vi "UAPublishNode.vi"(8 "error in (no error)":errorcluster, 9 "parent opcua path":string, 10 "OPC UA server refnum in":refnum<k21>, 11 "content":string) -> (0 "error out":errorcluster, 2 "OPC UA server refnum out":refnum<k21>)   [LabVIEW 2014, in "OPCUA XML(dev).lvlib"]
uses:
  OPCUA XML(dev).lvlib
  <vilib>/regexp/Match Regular Expression.xnode
  <vilib>/OPCUA/NI OPC UA Server.lvlib
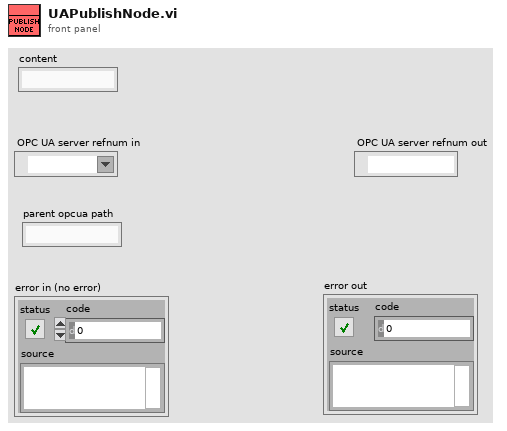
[diagram p1: front panel]
types:
  T1 = cluster{"name":string, "data type":u16, "access level":u16, "description":string}
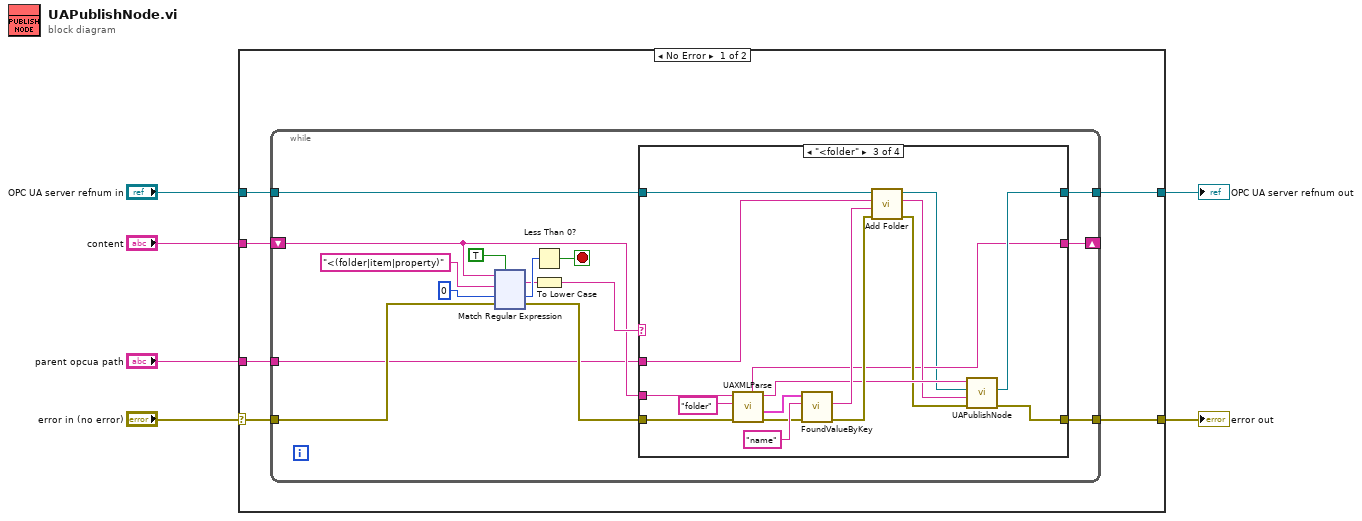
[diagram p0: block diagram]
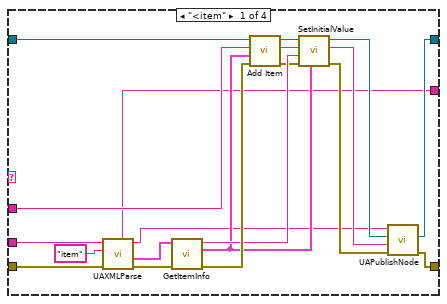
[diagram p2: hidden frame]
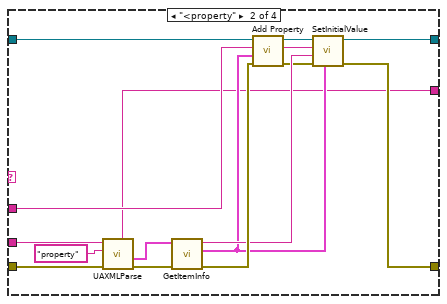
[diagram p3: hidden frame]
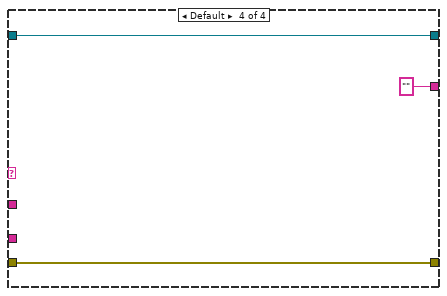
[diagram p4: hidden frame]
diagram:
  n1 = case shown="No Error" "error in (no error)" {
    selector: "error in (no error)" -> [w7 w199]
    tunnel: "content" -> [w12 _]
    tunnel: "OPC UA server refnum in" -> [w11 w198]
    tunnel: [w10 w199] -> w4
    tunnel: [w9 w198] -> w3
    tunnel: "parent opcua path" -> [w8 _]
    frame No Error {
      n2 = while {
        shift-right: [w13] -> _
        shift-left: w12 -> [w17]
        tunnel: [w15] -> w9
        tunnel: w11 -> [w16]
        tunnel: w7 -> [w22]
        tunnel: [w18] -> w10
        tunnel: w8 -> [w14]
        stop <- w23 stop-if-true
        n3 = xnode "Match Regular Expression"("input string"=w17, "regular expression"="<(folder|item|property)", "offset (0)"=0, "error in"=w22, "ignore case? (F)"=TRUE) -> ("whole match"=w21:string, "offset past match"=w24:i32, "error out"=w19:errorcluster)  [unwired: 1 in, 2 out]
        n4 = Less Than 0?(x=w24) -> (x < 0?=w23:bool)
        n5 = To Lower Case(string=w21) -> (all lower case string=w20:string)
        n6 = case shown="\"<folder\"" w20 {
          tunnel: w19 -> [w47 w63 w80 w82]
          tunnel: [w33 w50 w70 w82] -> w18
          tunnel: w17 -> [w46 w62 w79 _]
          tunnel: w16 -> [w43 w59 w77 w83]
          tunnel: [w30 w49 w69 w83] -> w15
          tunnel: w14 -> [w39 w55 w76 _]
          tunnel: [w28 w48 w65 "" ("after substring")] -> w13
          frame "<item" {
            n7 = call "UAXMLParse.vi"("error in (no error)"=w47, "label"="item", "string"=w46) -> ("error out"=w40:errorcluster, "keyValues"=w41:cluster{"key":string, "value":string}[], "content"=w29:string, "after substring"=w28:string)  [unwired: 3 in, 2 out]
            n8 = call "GetItemInfo.vi"("error in (no error)"=w40, "Array"=w41) -> ("error out"=w38:errorcluster, "item"=w36:T1, "Value"=w37:string)  [unwired: 7 in]
            n9 = call <vilib>:"Add Item.vi"("error in (no error)"=w38, "item"=w36, "parent folder path"=w39, "OPC UA server refnum in"=w43) -> ("error out"=w35:errorcluster, "item path"=w44:string, "OPC UA server refnum out"=w42:refnum<k21>)  [unwired: 4 in]
            n10 = call "SetInitialValue.vi"("item"=w36, "Error In"=w35, "value string"=w37, "node path"=w44, "OPC UA server refnum in"=w42) -> ("Error Out"=w34:errorcluster, "node path (dup)"=w32:string, "OPC UA server refnum out"=w31:refnum<k21>)  [unwired: 4 in]
            n11 = call "UAPublishNode.vi"("error in (no error)"=w34, "parent opcua path"=w32, "OPC UA server refnum in"=w31, "content"=w29) -> ("error out"=w33:errorcluster, "OPC UA server refnum out"=w30:refnum<k21>)  [unwired: 6 in]
          }
          frame "<property" {
            n12 = call "UAXMLParse.vi"("error in (no error)"=w63, "label"="property", "string"=w62) -> ("error out"=w56:errorcluster, "keyValues"=w57:cluster{"key":string, "value":string}[], "after substring"=w48:string)  [unwired: 3 in, 3 out]
            n13 = call "GetItemInfo.vi"("error in (no error)"=w56, "Array"=w57) -> ("error out"=w54:errorcluster, "item"=w52:T1, "Value"=w53:string)  [unwired: 7 in]
            n14 = call <vilib>:"Add Property.vi"("error in (no error)"=w54, "property"=w52, "item path"=w55, "OPC UA server refnum in"=w59) -> ("error out"=w51:errorcluster, "property path"=w60:string, "OPC UA server refnum out"=w58:refnum<k21>)  [unwired: 4 in]
            n15 = call "SetInitialValue.vi"("item"=w52, "Error In"=w51, "value string"=w53, "node path"=w60, "OPC UA server refnum in"=w58) -> ("Error Out"=w50:errorcluster, "OPC UA server refnum out"=w49:refnum<k21>)  [unwired: 4 in, 1 out]
          }
          frame "<folder" {
            n16 = call "UAXMLParse.vi"("error in (no error)"=w80, "label"="folder", "string"=w79) -> ("error out"=w73:errorcluster, "keyValues"=w75:cluster{"key":string, "value":string}[], "content"=w68:string, "after substring"=w65:string)  [unwired: 3 in, 2 out]
            n17 = call "FoundValueByKey.vi"("error in (no error)"=w73, "key"="name", "keyValues"=w75) -> ("error out"=w72:errorcluster, "value"=w71:string)  [unwired: 5 in, 2 out]
            n18 = call <vilib>:"Add Folder.vi"("error in (no error)"=w72, "folder name"=w71, "parent folder path"=w76, "OPC UA server refnum in"=w77) -> ("error out"=w67:errorcluster, "folder path"=w66:string, "OPC UA server refnum out"=w64:refnum<k21>)  [unwired: 4 in]
            n19 = call "UAPublishNode.vi"("error in (no error)"=w67, "parent opcua path"=w66, "OPC UA server refnum in"=w64, "content"=w68) -> ("error out"=w70:errorcluster, "OPC UA server refnum out"=w69:refnum<k21>)  [unwired: 6 in]
          }
          frame Default {
          }
        }
      }
    }
    frame Error {
    }
  }
  "error out" <- w4
  "OPC UA server refnum out" <- w3
